vi "Format Table Rows into Table.vi"(9 "Table Headers":string[](array[string]), 11 "Table Rows":string[](array[string])) -> (3 "Table Text":string)   [LabVIEW 2023, in "Confluence Formatting.lvlib"]
uses:
  Confluence Formatting.lvlib
  Types/Format Combo Box.ctl
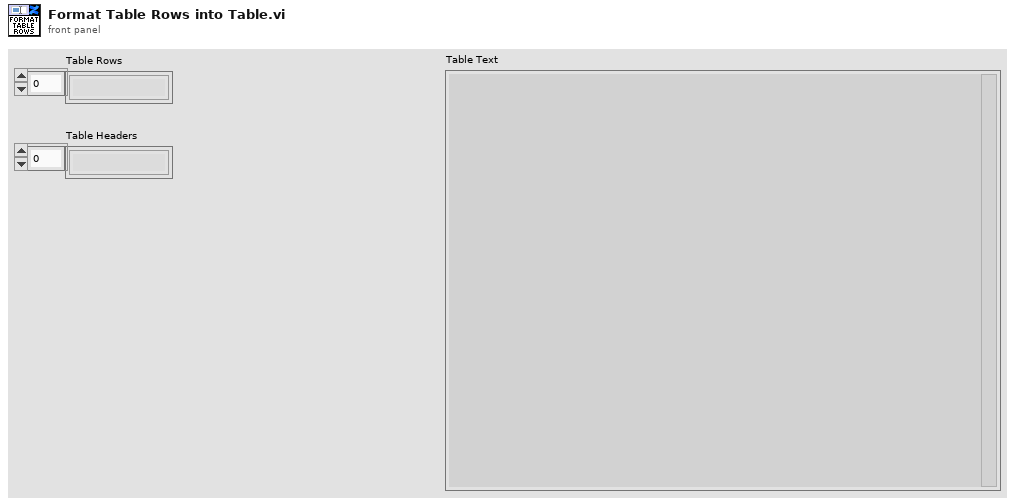
[diagram p1: front panel]
types:
  T1 = typedef "Confluence Formatting.lvlib/Format Combo Box.ctl" = string
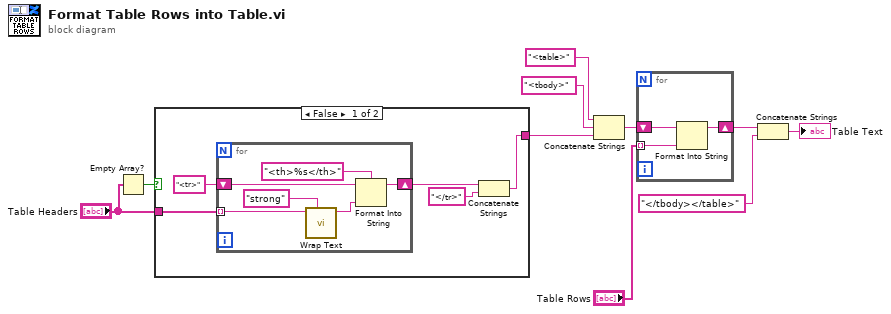
[diagram p0: block diagram]
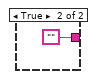
[diagram p2: hidden frame]
diagram:
  n1 = Empty Array?(array="Table Headers") -> (empty?=w4:bool)
  n2 = case shown="False" w4 {
    tunnel: "Table Headers" -> [w14 _]
    tunnel: [w11 ""] -> w2
    frame False {
      n3 = for {
        tunnel: w14 -> [w21] mode=indexing
        shift-right: [w16] -> w12
        shift-left: "<tr>" -> [w18]
        n4 = call "Wrap Text.vi"("Formatting"=T1 "strong", "String"=w21) -> ("Wrapped String"=w19:string)  [unwired: 8 in, 1 out]
        n5 = Format Into String(format string="<th>%s</th>", initial string=w18, w19) -> (resulting string=w16:string)  [unwired: 1 in, 1 out]
      }
      n6 = Concatenate Strings(w12, "</tr>" ("string")) -> (w11:string)
    }
    frame True {
    }
  }
  n7 = Concatenate Strings("<table>", "<tbody>" ("string"), w2) -> (w3:string)
  n8 = for {
    tunnel: "Table Rows" -> [w24] mode=indexing
    shift-right: [w23] -> w8
    shift-left: w3 -> [w25]
    n9 = Format Into String(initial string=w25, w24) -> (resulting string=w23:string)  [unwired: 2 in, 1 out]
  }
  n10 = Concatenate Strings(w8, "</tbody></table>" ("string")) -> (→"Table Text":string)
